vi "Test1000.vi"() -> ()   [LabVIEW 2016]
uses:
  Control/Coordinate.ctl
panel:
  in  "Est.Center":T1={"X"=717.7934, "Y"=883.43791, "Z"=0.0, "U"=0.0} {"U" format="%#.5g"; "X" format="%#.5g"; "Y" format="%#.5g"; "Z" format="%#.5g"}
  out "LaserCenter":T1 {"U" format="%#.5g"; "X" format="%#.5g"; "Y" format="%#.5g"; "Z" format="%#.5g"}
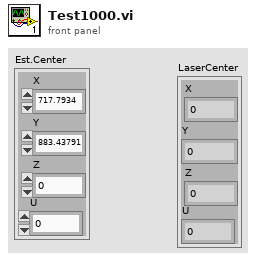
[diagram p1: front panel]
types:
  T1 = typedef "Coordinate.ctl" = cluster{"X":dbl, "Y":dbl, "Z":dbl, "U":dbl}
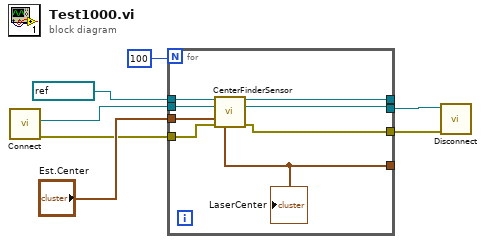
[diagram p0: block diagram]
diagram:
  n1 = call "Connect.vi"() -> ("error out"=w2:errorcluster, "controller"=w6:refnum<k24>)  [unwired: 10 in]
  n2 = for {
    N: 100 -> [_]
    tunnel: refnum<visa-resource-name> "COM4" ("VISA resource name") -> [w15]
    tunnel: w6 -> [w14]
    tunnel: "Est.Center" -> [w13]
    tunnel: [w12] -> _
    tunnel: [w11] -> w3
    tunnel: [w10] -> _
    tunnel: w2 -> [w9]
    tunnel: [w8] -> w1
    n3 = call "CenterFinderSensor.vi"("VISA resource name"=w15, "controller in"=w14, "Est.Center"=w13, "error in (no error)"=w9) -> ("VISA resource name out"=w12:refnum<visa-resource-name>, "controller out"=w11:refnum<k24>, "LaserCenter"=w10:T1, "error out 2"=w8:errorcluster)  [unwired: 6 in, 2 out]
    "LaserCenter" <- w10
  }
  n4 = call "Disconnect.vi"("error in (no error)"=w1, "controller"=w3) -> ()  [unwired: 9 in, 1 out]
